vi "RSNRPZ Get Sensor Name.vi"(8 "error in (no error)":errorcluster, 9 "Max Length (10)":u32=10, 10 "Channel (1)":i32=1, 11 "VISA session":refnum<visa-resource-name> caption="VISA resource name") -> (0 "error out":errorcluster, 2 "Name":string, 3 "dup VISA session":refnum<visa-resource-name> caption="VISA resource name")   [LabVIEW 2010]
doc: "This VI returns the sensor name.\n\nRemote-control command(s):\nSENS:POW:TSL:AVG:COUN"
uses:
  rsnrpz_32.dll
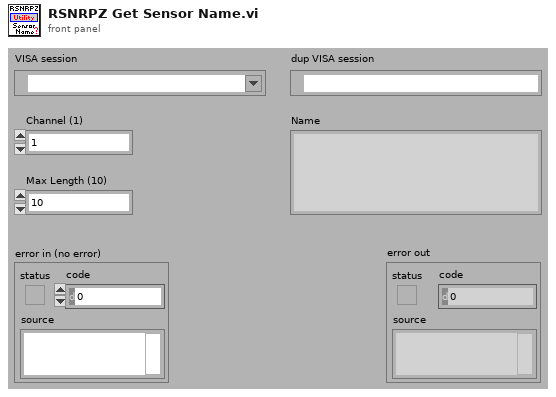
[diagram p1: front panel]
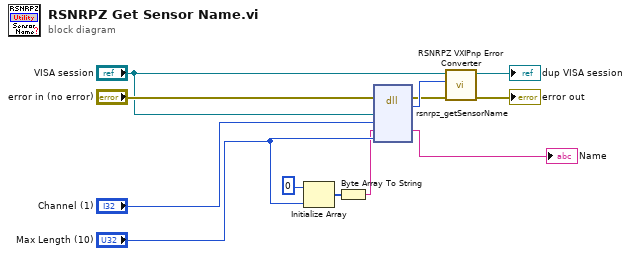
[diagram p0: block diagram]
diagram:
  n1 = Initialize Array(u8 0 ("element"), "Max Length (10)") -> (w7:u8[])
  n2 = Byte Array To String(unsigned byte array=w7) -> (string=w8:string)
  n3 = dll-call lib="rsnrpz_32.dll" fn="rsnrpz_getSensorName"(error in="error in (no error)", "Instrument Handle"="VISA session", "Channel"="Channel (1)", "Name"=w8, "Max Length"="Max Length (10)") -> (error out=w5:errorcluster, w9:i32, "Name"=→"Name":string)  [unwired: 5 in, 1 out]
  n4 = call <instrlib>:"RSNRPZ VXIPnp Error Converter.vi"("error in"=w5, "VXIPnp error code"=w9, "VISA session"="VISA session") -> ("error out"=→"error out":errorcluster, "dup VISA session"=→"dup VISA session":refnum<visa-resource-name>)  [unwired: 7 in]
